vi "Tosca-Remap Digital Inputs.vi"(0 "Events In":T2[](array[typedef]), 7 "Flags":T1[](array[typedef]), 11 "error in (no error)":errorcluster) -> (4 "Events out":T2[](array[typedef]), 15 "error out":errorcluster)   [LabVIEW 2020]
uses:
  Digital Input VIs/Tosca-Input Event.ctl
  Digital Input VIs/Tosca-Input Criterion.ctl
  epl-vi-lib/Utility VIs/Type Defs/Logic State.ctl
  Typedefs/Tosca-Accumulator.ctl
  Typedefs/Tosca-Flag.ctl
  Tosca-Globals.vi
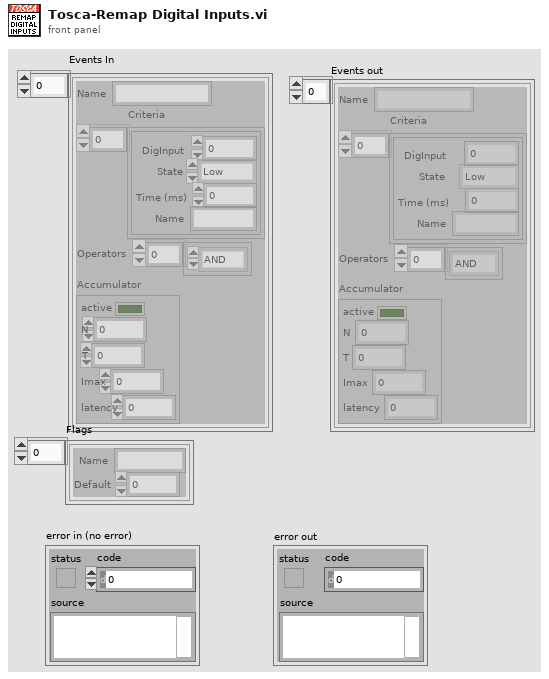
[diagram p1: front panel]
types:
  T1 = typedef "Tosca-Flag.ctl" = cluster{"Name":string, "Default":i32}
  T2 = typedef "Tosca-Input Event.ctl" = cluster{"Name":string, "Criteria":T3[], "Operators":enum16{"AND", "OR"}[], "Accumulator":T5}
  T3 = typedef "Tosca-Input Criterion.ctl" = cluster{"DigInput":i32, "State":T4, "Time (ms)":i32, "Name":string}
  T4 = typedef "Logic State.ctl" = enum16{"Low", "High", "Rising", "Falling"}
  T5 = typedef "Tosca-Accumulator.ctl" = cluster{"active":bool, "N":i32, "T":dbl, "Imax":dbl, "latency":dbl}
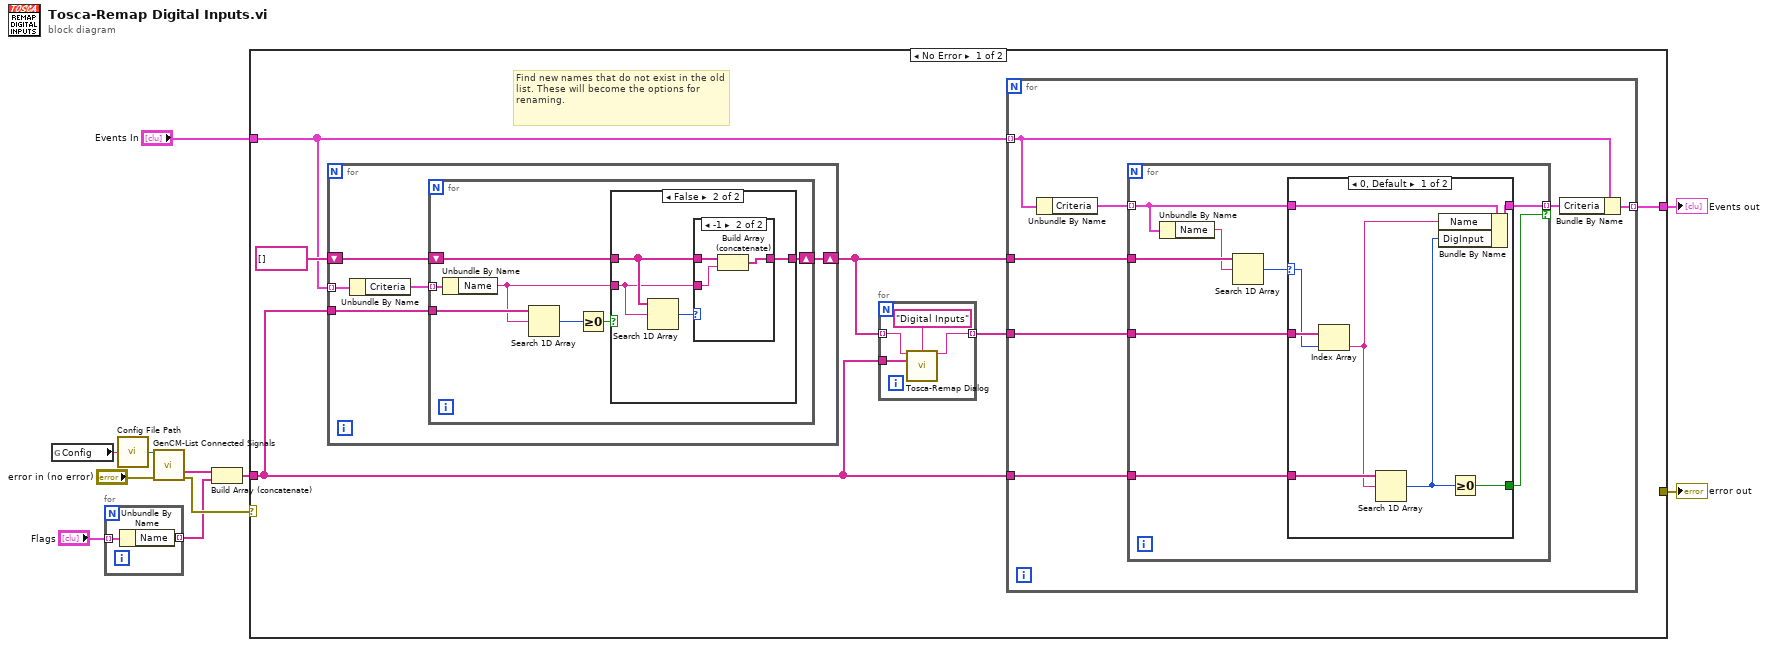
[diagram p0: block diagram]
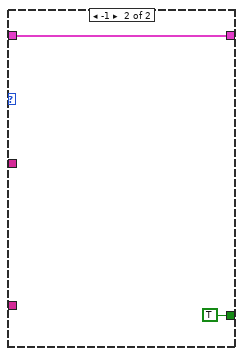
[diagram p2: hidden frame]
diagram:
  n1 = global read "Tosca-Globals.vi" "Config"() -> (w1:string)
  n2 = for {
    tunnel: "Flags" -> [w13] mode=indexing
    tunnel: [w12] -> w2 mode=indexing
    n3 = Unbundle By Name(w13) -> ("Name"=w12:string)
  }
  n4 = call "Config File Path.vi"("AppName"=w1) -> ("Default config file name"=w9:path)
  n5 = call "GenCM-List Connected Signals.vi"("Path"=w9, "error in (no error)"="error in (no error)") -> ("Digital Inputs"=w4:string[], "error out"=w7:errorcluster)  [unwired: 9 in, 3 out]
  n6 = Build Array (concatenate)(w4, w2) -> (w3:string[])
  n7 = case shown="No Error" w7 {
    selector: w7 -> [_ w71]
    tunnel: [_ w71] -> w11
    tunnel: "Events In" -> [w18 w70]
    tunnel: w3 -> [w14 _]
    tunnel: [w15 w70] -> w6
    frame No Error {
      # "Find new names that do not exist in the old list. These will become the options for renaming."
      n8 = for {
        tunnel: w18 -> [w48] mode=indexing
        shift-right: [w45] -> w17
        shift-left: string[] [] -> [w46]
        tunnel: w14 -> [w49]
        n9 = Unbundle By Name(w48) -> ("Criteria"=w47:T3[])
        n10 = for {
          tunnel: w47 -> [w53] mode=indexing
          shift-right: [w50] -> w45
          shift-left: w46 -> [w51]
          tunnel: w49 -> [w54]
          n11 = Unbundle By Name(w53) -> ("Name"=w52:string)
          n12 = Search 1D Array(1D array=w54, element=w52) -> (index of element=w55:i32)  [unwired: 1 in]
          n13 = Greater Or Equal To 0?(x=w55) -> (x >= 0?=w56:bool)
          n14 = case shown="False" w56 {
            tunnel: w52 -> [_ w59]
            tunnel: w51 -> [w57 w61]
            tunnel: [w57 w58] -> w50
            frame True {
            }
            frame False {
              n15 = Search 1D Array(1D array=w61, element=w59) -> (index of element=w60:i32)  [unwired: 1 in]
              n16 = case shown="-1" w60 {
                tunnel: w61 -> [w62 w65]
                tunnel: w59 -> [_ w63]
                tunnel: [w62 w64] -> w58
                frame 0, Default {
                }
                frame -1 {
                  n17 = Build Array (concatenate)(w65, w63) -> (w64:string[])
                }
              }
            }
          }
        }
      }
      n18 = for {
        tunnel: [w68] -> w16 mode=indexing
        tunnel: w17 -> [w67] mode=indexing
        tunnel: w14 -> [w69]
        n19 = call "Tosca-Remap Dialog.vi"("Old Name In"=w67, "Type"="Digital Inputs", "New Names"=w69) -> ("Old Name Out"=w68:string)  [unwired: 10 in, 2 out]
      }
      n20 = for {
        tunnel: w18 -> [w22] mode=indexing
        tunnel: w17 -> [w25]
        tunnel: w16 -> [w24]
        tunnel: w14 -> [w23]
        tunnel: [w20] -> w15 mode=indexing
        n21 = Unbundle By Name(w22) -> ("Criteria"=w26:T3[])
        n22 = for {
          tunnel: w26 -> [w29] mode=indexing
          tunnel: w25 -> [w34]
          tunnel: w24 -> [w30]
          tunnel: [w31] -> w21 mode=indexing if=w27
          tunnel: w23 -> [w28]
          n23 = Unbundle By Name(w29) -> ("Name"=w33:string)
          n24 = Search 1D Array(1D array=w34, element=w33) -> (index of element=w32:i32)  [unwired: 1 in]
          n25 = case shown="0, Default" w32 {
            selector: w32 -> [w41 _]
            tunnel: [w39 w44] -> w31
            tunnel: w30 -> [w42 _]
            tunnel: w29 -> [w40 w44]
            tunnel: w28 -> [w38 _]
            tunnel: [w35 TRUE] -> w27
            frame 0, Default {
              n26 = Index Array(array=w42, index=w41) -> (element=w37:string)
              n27 = Search 1D Array(1D array=w38, element=w37) -> (index of element=w36:i32)  [unwired: 1 in]
              n28 = Bundle By Name(cluster=w40, "Name"=w37, "DigInput"=w36) -> (w39:T3)
              n29 = Greater Or Equal To 0?(x=w36) -> (x >= 0?=w35:bool)
            }
            frame -1 {
            }
          }
        }
        n30 = Bundle By Name(cluster=w22, "Criteria"=w21) -> (w20:T2)
      }
    }
    frame Error {
    }
  }
  "error out" <- w11
  "Events out" <- w6
